vi "Modbus Master.vi"(0 "starting address":u16 caption="起始地址", 1 "error in":errorcluster, 5 "holding register values":u16[](array[numeric]) caption="写入保持寄存器的值", 9 "读取写入选择":string(combo), 11 "Unit ID":u8=1) -> (3 "error out":errorcluster, 4 "仪器状态":u16[](array[numeric]), 6 "试剂余量":u16[](array[numeric]), 10 "各参数测量间隔":u16[](array[numeric]), 14 "校准点信息":u16[](array[numeric]), 15 "关键参数":u16[](array[numeric]))   [LabVIEW 2016, in "数据传输系统-03.lvlib"]
uses:
  <vilib>/NI/Modbus Library/API/Modbus API.lvclass/Modbus API.ctl
  <vilib>/NI/Modbus Library/Transmission Data Unit/Transmission Data Unit.lvclass/Transmission Data Unit.ctl
  <vilib>/NI/Modbus Library/API/Master/Set Unit ID.vi
  <vilib>/NI/Modbus Library/Transmission Data Unit/Write Unit ID.vi
  <vilib>/NI/Modbus Library/API/Read Transmission Data Unit.vi
  <vilib>/NI/Modbus Library/API/Write Transmission Data Unit.vi
  <vilib>/NI/Modbus Library/API/master/Modbus Master.lvclass
  D:/Program Files (x86)/National Instruments/LabVIEW 2016/vi.lib/NI/Modbus Library/API/Modbus API.lvclass
  <vilib>/NI/Modbus Library/API/Wrapper/Create TCP Master.vi
  <vilib>/NI/Modbus Library/API/Modbus API.lvclass
  <vilib>/NI/Modbus Library/API/Wrapper/API Main.lvlib
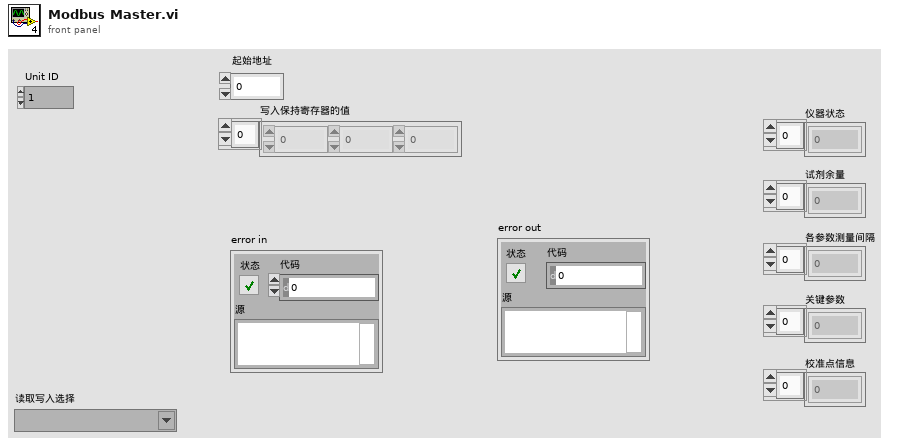
[diagram p1: front panel]
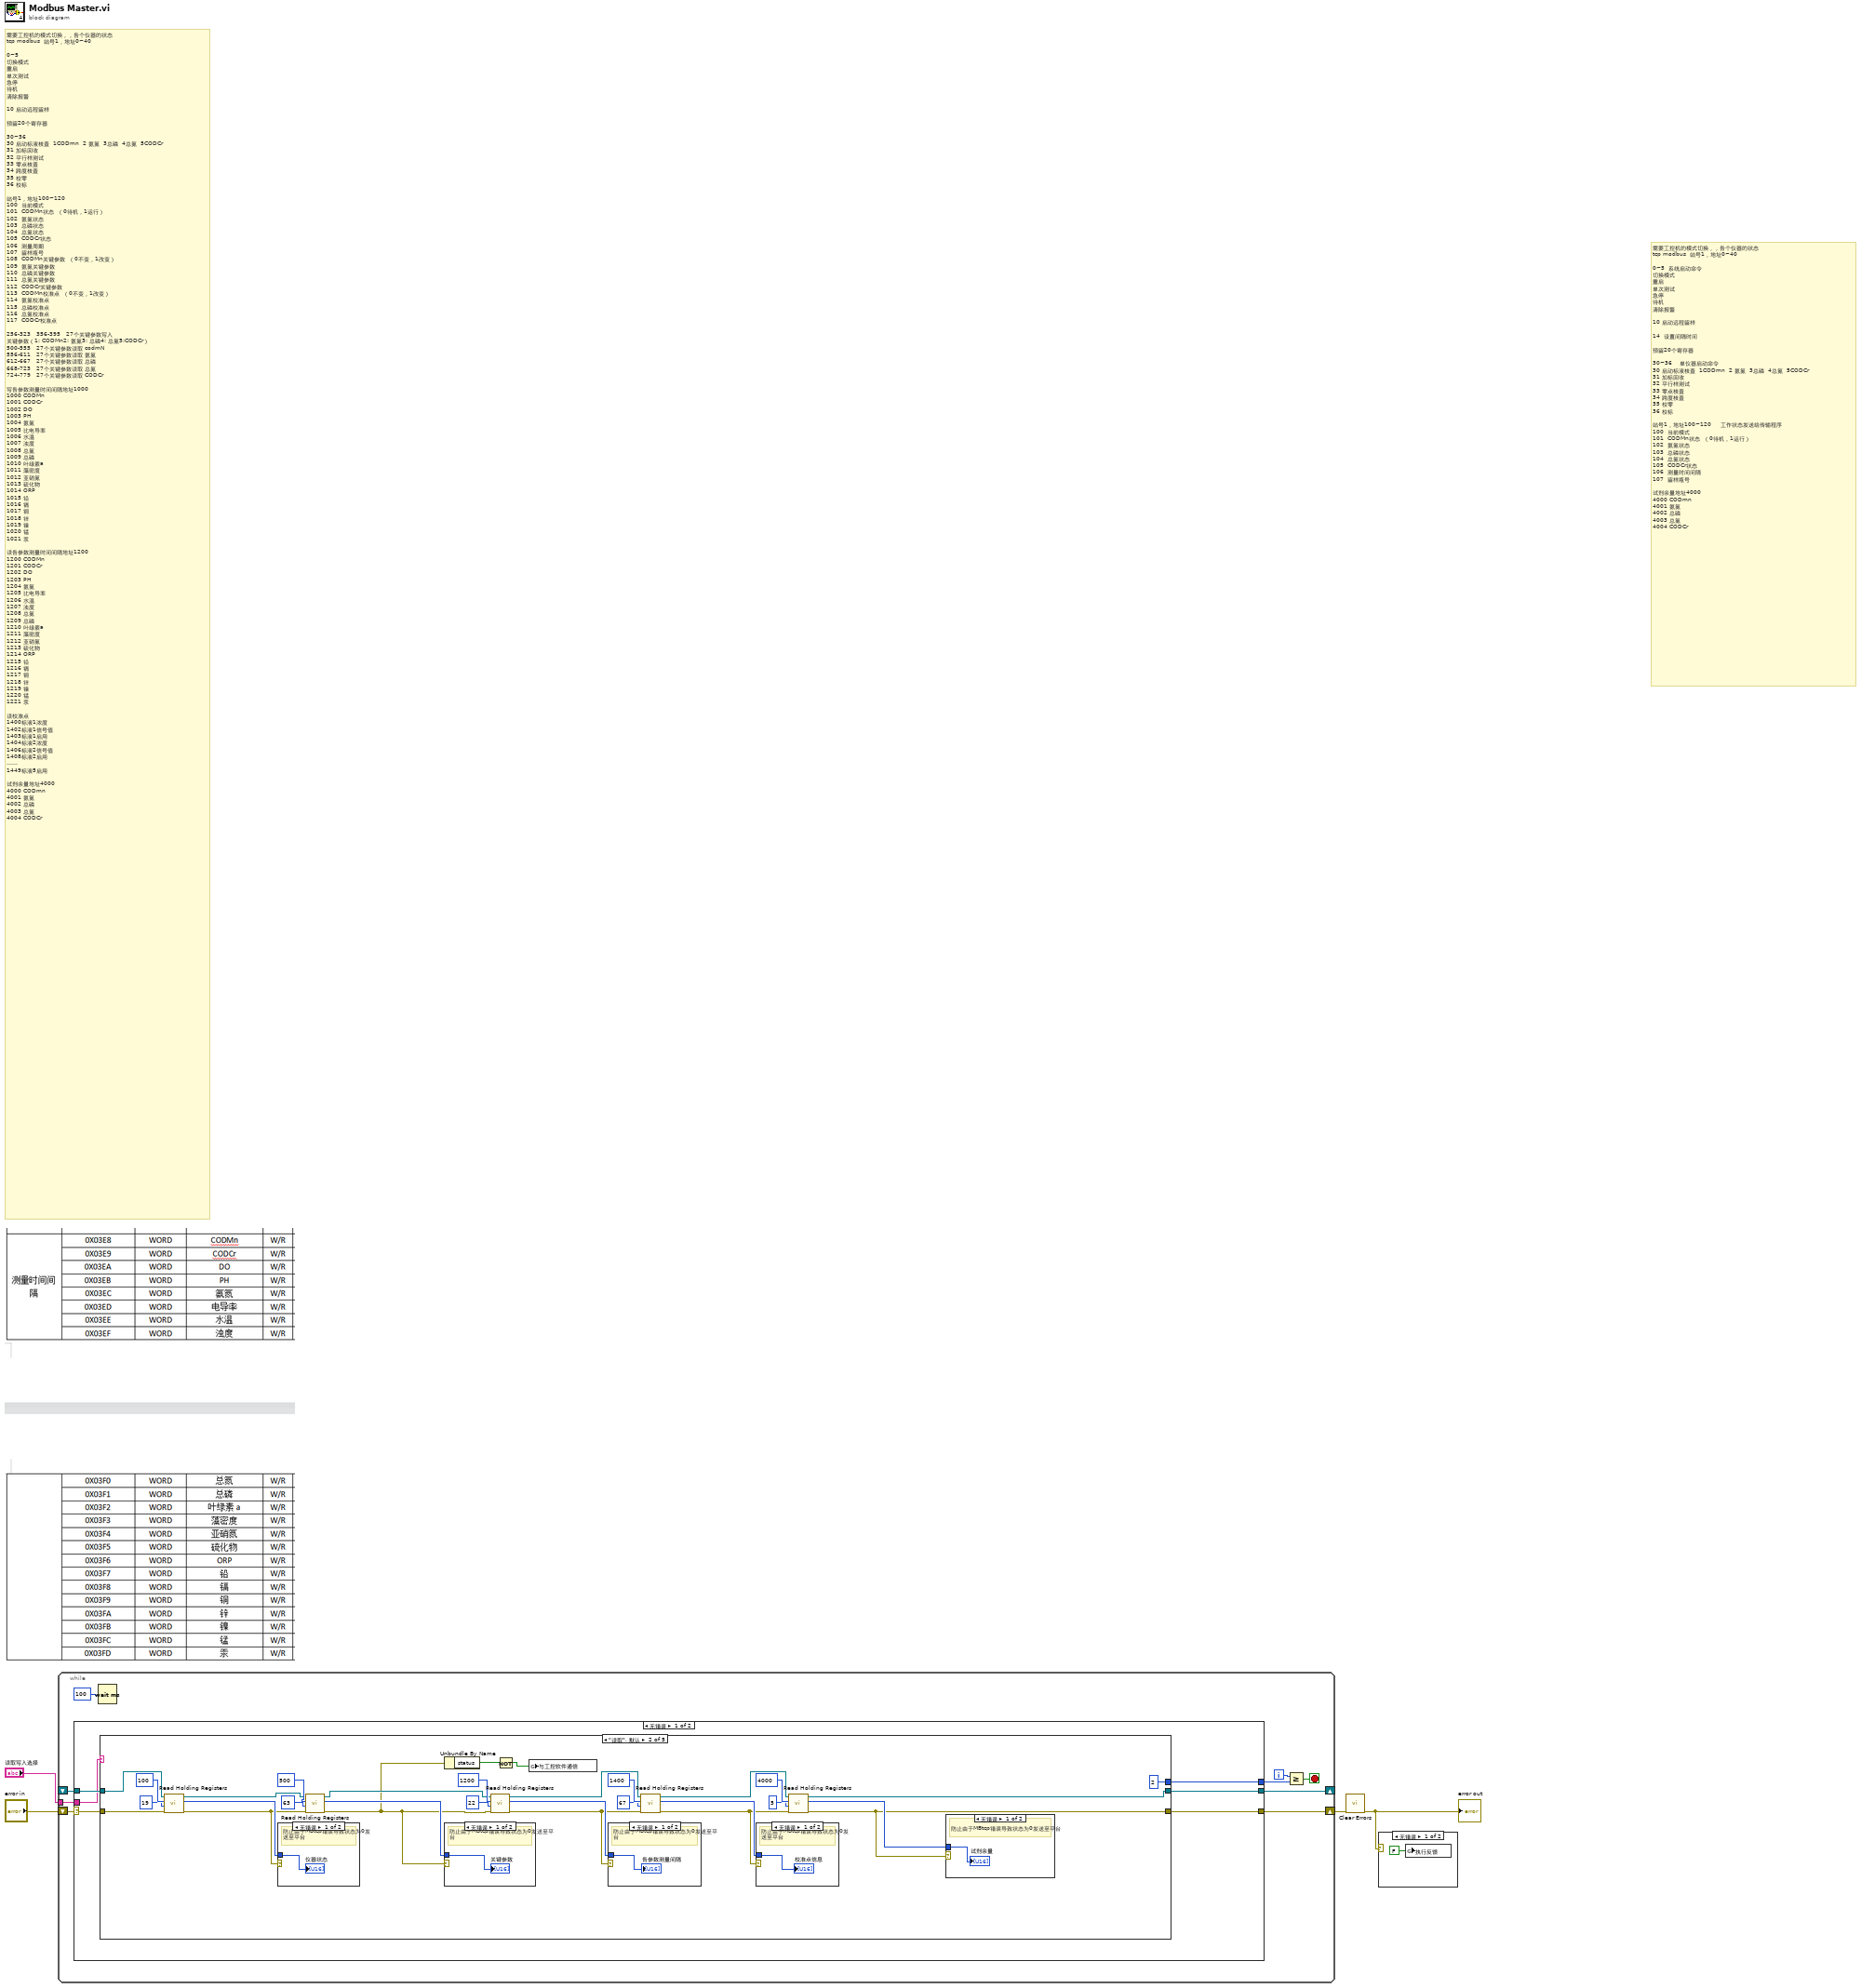
[diagram p0: block diagram]
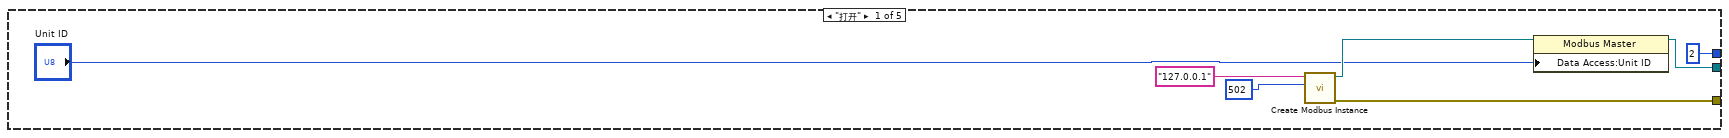
[diagram p3: hidden frame]
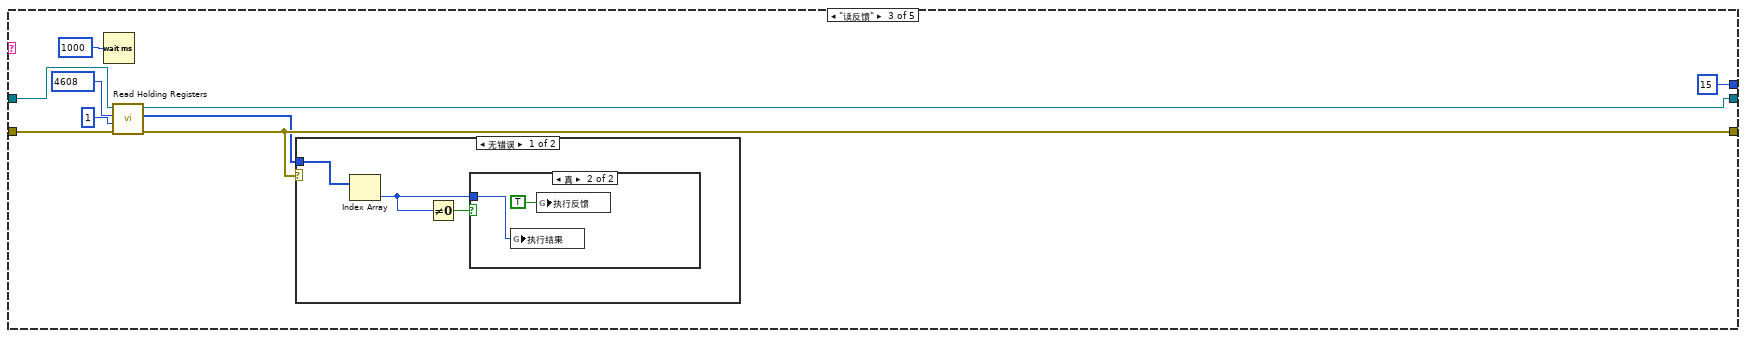
[diagram p9: hidden frame]
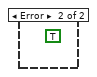
[diagram p11: hidden frame]
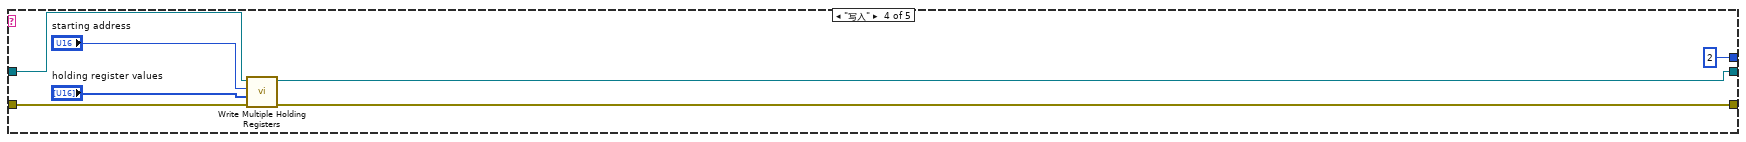
[diagram p12: hidden frame]
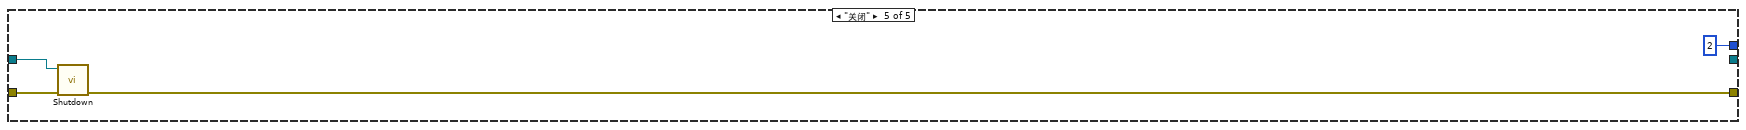
[diagram p13: hidden frame]
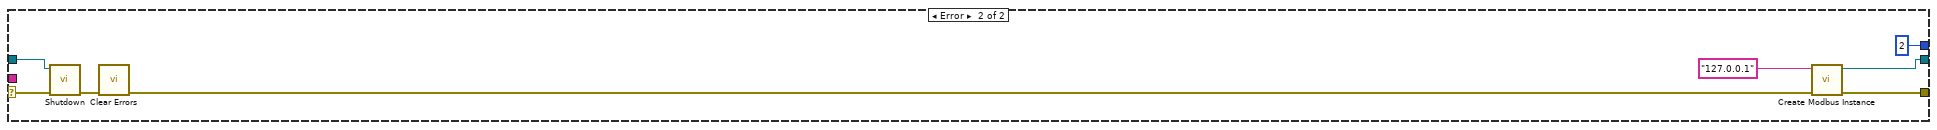
[diagram p14: hidden frame]
diagram:
  # "需要工控机的模式切换，，各个仪器的状态\ntcp modbus  站号1，地址0~40\n\n0~5  系统启动命令\n切换模式\n重启\n单次测试\n急停\n待机\n清除报警\n\n10 启动远程留样\n\n14  设置间隔时间\n\n预留20个寄存器\n\n30~36    单仪器启动命令\n30 启动标液核查  1CODmn  2 氨氮  3总磷  4总氮  5CODCr\n31 加标回收\n32 平行样测试\n33 零点核查\n34 跨度核查\n35 校零\n36 校标\n\n站号1，地址100~120     工作状态发送给传输程序\n100  当前模式\n101  CODMn状态  （0待机，1运行）\n102  氨氮状态\n103  总磷状态\n104  总氮状态\n105  CODCr状态\n106  测量时间间隔\n107  留样瓶号\n\n试剂余量地址4000\n4000 CODmn\n4001 氨氮\n4002 总磷\n4003 总氮\n4004 CODCr"
  # "需要工控机的模式切换，，各个仪器的状态\ntcp modbus  站号1，地址0~40\n\n0~5\n切换模式\n重启\n单次测试\n急停\n待机\n清除报警\n\n10 启动远程留样\n\n预留20个寄存器\n\n30~36\n30 启动标液核查  1CODmn  2 氨氮  3总磷  4总氮  5CODCr\n31 加标回收\n32 平行样测试\n33 零点核查\n34 跨度核查\n35 校零\n36 校标\n\n站号1，地址100~120\n100  当前模式\n101  CODMn状态  （0待机，1运行）\n102  氨氮状态\n103  总磷状态\n104  总氮状态\n105  CODCr状态\n106  测量周期\n107  留样瓶号\n108  CODMn关键参数  （0不变，1改变）\n109  氨氮关键参数\n110  总磷关键参数\n111  总氮关键参数\n112  CODCr关键参数\n113  CODMn校准点  （0不变，1改变）\n114  氨氮校准点\n115  总磷校准点\n116  总氮校准点\n117  CODCr校准点\n\n256-323   356-395   27个关键参数写入\n关键参数（1: CODMn2: 氨氮3: 总磷4: 总氮5:CODCr） \n500-555   27个关键参数读取 codmN\n556-611   27个关键参数读取 氨氮\n612-667   27个关键参数读取 总磷\n668-723   27个关键参数读取 总氮\n724-779   27个关键参数读取 CODCr\n\n写各参数测量时间间隔地址1000\n1000 CODMn\n1001 CODCr\n1002 DO\n1003 PH\n1004 氨氮\n1005 比电导率\n1006 水温\n1007 浊度\n1008 总氮\n1009 总磷\n1010 叶绿素a\n1011 藻密度\n1012 亚硝氮\n1013 硫化物\n1014 ORP\n1015 铅\n1016 镉\n1017 铜\n1018 锌\n1019 镍\n1020 锰\n1021 汞\n\n读各参数测量时间间隔地址1200\n1200 CODMn\n1201 CODCr\n1202 DO\n1203 PH\n1204 氨氮\n1205 比电导率\n1206 水温\n1207 浊度\n1208 总氮\n1209 总磷\n1210 叶绿素a\n1211 藻密度\n1212 亚硝氮\n1213 硫化物\n1214 ORP\n1215 铅\n1216 镉\n1217 铜\n1218 锌\n1219 镍\n1220 锰\n1221 汞\n\n读校准点\n1400标液1浓度\n1402标液1信号值\n1403标液1启用\n1404标液2浓度\n1406标液2信号值\n1408标液2启用\n......\n1449标液5启用\n\n试剂余量地址4000\n4000 CODmn\n4001 氨氮\n4002 总磷\n4003 总氮\n4004 CODCr"
  n1 = while {
    shift-right: [w7] -> w2
    shift-left: "error in" -> [w11]
    shift-right: [w12] -> _
    shift-left: _ -> [w13]
    tunnel: "读取写入选择" -> [w8]
    i -> [w9]
    stop <- w6 stop-if-true
    n2 = case shown="无错误" w11 {
      selector: w11 -> [w16 w88]
      tunnel: w13 -> [w19 w90]
      tunnel: [w18 w92] -> w12
      tunnel: [w17 w91] -> w7
      tunnel: w8 -> [w15 _]
      tunnel: [w14 2 ("y")] -> w5
      frame No Error {
        n3 = case shown="\"读取\", 默认" w15 {
          tunnel: w19 -> [_ w56 w68 w82 w86]
          tunnel: [w23 w35 w66 w81 _] -> w18
          tunnel: [w22 w45 w65 w80 w84] -> w17
          tunnel: w16 -> [_ w55 w67 w79 w85]
          tunnel: [2 ("y") 2 ("y") 15 ("y") 2 ("y") 2 ("y")] -> w14
          frame "打开" {
            n4 = call-poly <vilib>:"Create Modbus Instance.vi"("port (502)"=u16 502, "address"="127.0.0.1") -> ("error out"=w22:errorcluster, "TCP master instance"=w26:refnum<class "Modbus Master.lvclass">)  [unwired: 8 in]
            n5 = property class="Modbus Master"(reference=w26, "Data Access:Unit ID"="Unit ID") -> (reference out=w23:refnum<class "Modbus Master.lvclass">)  [unwired: 1 in, 1 out]
          }
          frame "读取", Default {
            n6 = call-dynamic "Read Holding Registers.vi"("error in"=w55, "number of inputs"=u16 19 ("number of holding registers"), "starting address"=u16 100, "Modbus instance in"=w56) -> ("error out"=w36:errorcluster, "register values"=w52:u16[], "Modbus instance out"=w39:refnum<class "Modbus API.lvclass">)  [unwired: 5 in]
            n7 = case shown="无错误" w36 {
              tunnel: w52 -> [w61 _]
              frame No Error {
                # "防止由于MBtcp错误导致状态为0发送至平台"
                "仪器状态" <- w61
              }
              frame Error {
              }
            }
            n8 = call-dynamic "Read Holding Registers.vi"("error in"=w36, "number of inputs"=u16 63 ("number of holding registers"), "starting address"=u16 500, "Modbus instance in"=w39) -> ("error out"=w27:errorcluster, "register values"=w37:u16[], "Modbus instance out"=w38:refnum<class "Modbus API.lvclass">)  [unwired: 5 in]
            n9 = Unbundle By Name(w27) -> ("status"=w50:bool)
            n10 = case shown="无错误" w27 {
              tunnel: w37 -> [w58 _]
              frame No Error {
                # "防止由于MBtcp错误导致状态为0发送至平台"
                "关键参数" <- w58
              }
              frame Error {
              }
            }
            n11 = call-dynamic "Read Holding Registers.vi"("error in"=w27, "number of inputs"=u16 22 ("number of holding registers"), "starting address"=u16 1200, "Modbus instance in"=w38) -> ("error out"=w31:errorcluster, "register values"=w42:u16[], "Modbus instance out"=w32:refnum<class "Modbus API.lvclass">)  [unwired: 5 in]
            n12 = Not(x=w50) -> (.not. x?=w49:bool)
            n13 = global write "全局1.vi" "与工控软件通信"(w49) -> ()
            n14 = case shown="无错误" w31 {
              tunnel: w42 -> [w59 _]
              frame No Error {
                # "防止由于MBtcp错误导致状态为0发送至平台"
                "各参数测量间隔" <- w59
              }
              frame Error {
              }
            }
            n15 = call-dynamic "Read Holding Registers.vi"("error in"=w31, "number of inputs"=u16 67 ("number of holding registers"), "starting address"=u16 1400, "Modbus instance in"=w32) -> ("error out"=w28:errorcluster, "register values"=w30:u16[], "Modbus instance out"=w29:refnum<class "Modbus API.lvclass">)  [unwired: 5 in]
            n16 = case shown="无错误" w28 {
              tunnel: w30 -> [w57 _]
              frame No Error {
                # "防止由于MBtcp错误导致状态为0发送至平台"
                "校准点信息" <- w57
              }
              frame Error {
              }
            }
            n17 = call-dynamic "Read Holding Registers.vi"("error in"=w28, "number of inputs"=u16 5 ("number of holding registers"), "starting address"=u16 4000, "Modbus instance in"=w29) -> ("error out"=w45:errorcluster, "register values"=w46:u16[], "Modbus instance out"=w35:refnum<class "Modbus API.lvclass">)  [unwired: 5 in]
            n18 = case shown="无错误" w45 {
              tunnel: w46 -> [w60 _]
              frame No Error {
                # "防止由于MBtcp错误导致状态为0发送至平台"
                "试剂余量" <- w60
              }
              frame Error {
              }
            }
          }
          frame "读反馈" {
            n19 = Wait (ms)(milliseconds to wait=u32 1000 ("等待时间（毫秒）")) -> ()  [unwired: 1 out]
            n20 = call-dynamic "Read Holding Registers.vi"("error in"=w67, "number of inputs"=u16 1 ("number of holding registers"), "starting address"=u16 4608, "Modbus instance in"=w68) -> ("error out"=w65:errorcluster, "register values"=w64:u16[], "Modbus instance out"=w66:refnum<class "Modbus API.lvclass">)  [unwired: 5 in]
            n21 = case shown="无错误" w65 {
              tunnel: w64 -> [w73 _]
              frame No Error {
                n22 = Index Array(array=w73) -> (element=w72:u16)  [unwired: 1 in]
                n23 = Not Equal To 0?(x=w72) -> (x != 0?=w71:bool)
                n24 = case shown="真" w71 {
                  tunnel: w72 -> [_ w74]
                  frame False {
                  }
                  frame True {
                    n25 = global write "全局 反控命令枚举.vi" "执行结果"(w74) -> ()
                    n26 = global write "全局 反控命令枚举.vi" "执行反馈"(TRUE ("执行反馈")) -> ()
                  }
                }
              }
              frame Error {
                (unwired) TRUE
              }
            }
          }
          frame "写入" {
            n27 = call-dynamic "Write Multiple Holding Registers.vi"("error in"=w79, "registers to write"="holding register values", "starting address"="starting address", "Modbus instance in"=w82) -> ("error out"=w80:errorcluster, "Modbus instance out"=w81:refnum<class "Modbus API.lvclass">)  [unwired: 6 in]
          }
          frame "关闭" {
            n28 = call-dynamic "Shutdown.vi"("error in"=w85, "Modbus instance in"=w86) -> ("error out"=w84:errorcluster)  [unwired: 9 in]
          }
        }
      }
      frame Error {
        n29 = call-dynamic "Shutdown.vi"("error in"=w88, "Modbus instance in"=w90) -> ("error out"=w89:errorcluster)  [unwired: 9 in]
        n30 = call <vilib>:"Clear Errors.vi"("error in (no error)"=w89) -> ("error out"=w93:errorcluster)  [unwired: 5 in, 1 out]
        n31 = call-poly <vilib>:"Create Modbus Instance.vi"("error in"=w93, "address"="127.0.0.1") -> ("error out"=w91:errorcluster, "TCP master instance"=w92:refnum<class "Modbus Master.lvclass">)  [unwired: 8 in]
      }
    }
    n32 = Wait (ms)(milliseconds to wait=u32 100 ("等待时间（毫秒）")) -> ()  [unwired: 1 out]
    n33 = Greater Or Equal?(x=w9, y=w5) -> (x >= y?=w6:bool)
  }
  n34 = call <vilib>:"Clear Errors.vi"("error in (no error)"=w2) -> ("error out"=w1:errorcluster)  [unwired: 5 in, 1 out]
  "error out" <- w1
  n35 = case shown="无错误" w1 {
    frame No Error {
      n36 = global write "全局 反控命令枚举.vi" "执行反馈"(FALSE ("执行反馈")) -> ()
    }
    frame Error {
    }
  }
